vi "Pulses to rad per sec.vi"(11 "Encoder pulses":dbl) -> (1 "RPM":dbl, 2 "Deg/s 2":dbl, 3 "Rad/s":dbl)   [LabVIEW 2016]
doc: "Takes two inputs,"
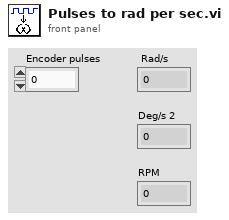
[diagram p1: front panel]
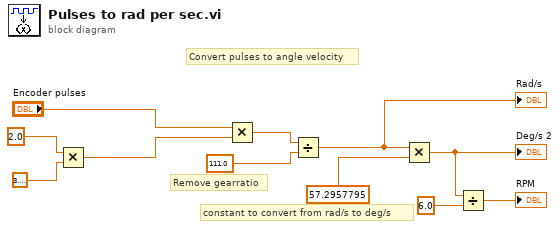
[diagram p0: block diagram]
diagram:
  # "Remove gearratio"
  # "constant to convert from rad/s to deg/s"
  # "Convert pulses to angle velocity"
  n1 = Multiply(x=2.0, y=3.141592653589793) -> (x*y=w9:dbl)
  n2 = Multiply(x="Encoder pulses", y=w9) -> (x*y=w8:dbl)
  n3 = Divide(x=w8, y=111.0) -> (x/y=w4:dbl)
  "Rad/s" <- w4
  n4 = Multiply(x=w4, y=57.2957795) -> (x*y=w1:dbl)
  "Deg/s 2" <- w1
  n5 = Divide(x=w1, y=6.0) -> (x/y=→"RPM":dbl)
